vi "DownloadPackageFromNevstopFTP.vi"(8 "error in (no error)":errorcluster, 11 "CommandLine":string[](array[string])) -> (0 "error out":errorcluster, 2 "test details":string, 3 "output to action":string)   [LabVIEW 2014]
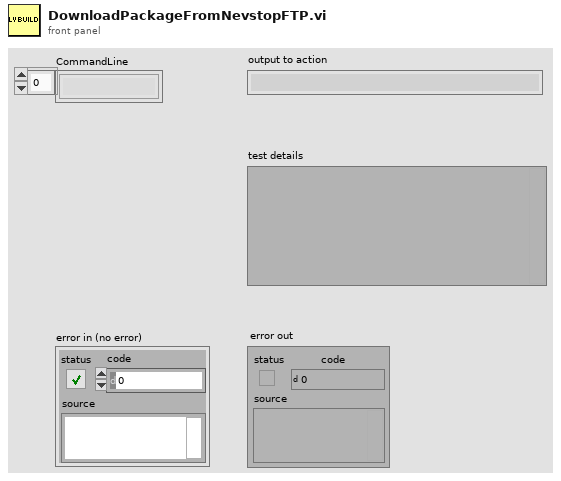
[diagram p1: front panel]
types:
  T1 = cluster{"address":string, "remote port (21)":u16, "userName":string, "passWord":string}
  T2 = typedef "FTP.lvlib/FTP.lvclass/Dir-File Info.ctl" = cluster{"Name":string, "Modify Timestamp":timestamp, "Dir-File Type":T3, "Unique Id":string, "Permissions":string, "Unix Mode":u16, "Owner":string, "Group":string, "FileSize":i64}
  T3 = typedef "FTP.lvlib/FTP.lvclass/Dir-File Type.ctl" = enum16{"File", "Listed Directory", "Parent Directory", "Directory", "Unknown"}
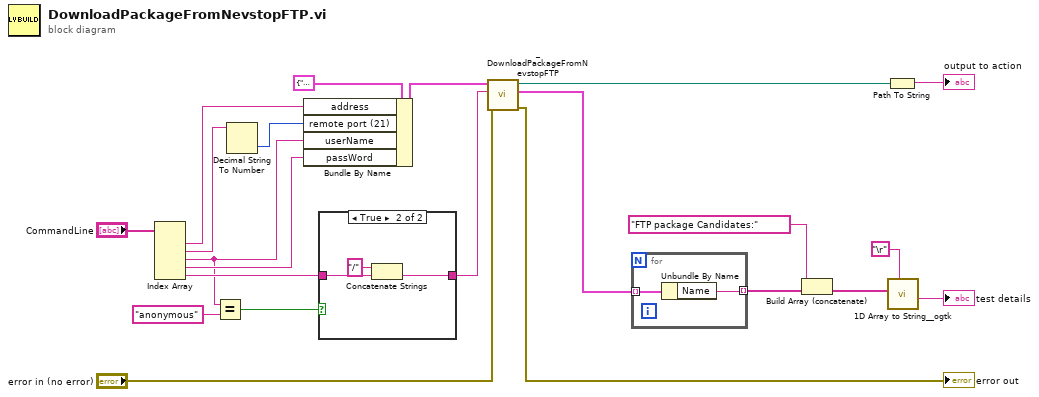
[diagram p0: block diagram]
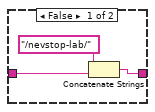
[diagram p2: hidden frame]
diagram:
  n1 = Index Array(array="CommandLine") -> (element #1=w16:string, element #2=w15:string, element #3=w3:string, element #4=w13:string, element #5=w12:string)  [unwired: 5 in]
  n2 = Equal?(x=w3, y="anonymous") -> (x = y?=w1:bool)
  n3 = Decimal String To Number(string=w15) -> (number=w14:i32)  [unwired: 2 in, 1 out]
  n4 = Bundle By Name(cluster=T1 {"address"="vipm.nevstop.top", "remote port (21)"=1986, "userName"="", "passWord"=""} ("ftp"), "address"=w16, "remote port (21)"=w14, "userName"=w3, "passWord"=w13) -> (w17:T1)
  n5 = case shown="True" w1 {
    tunnel: w12 -> [w25 w28]
    tunnel: [w23 w27] -> w11
    frame False {
      n6 = Concatenate Strings("/nevstop-lab/" ("RemoteDirectory"), w25) -> (w23:string)
    }
    frame True {
      n7 = Concatenate Strings("/" ("string"), w28) -> (w27:string)
    }
  }
  n8 = call "_DownloadPackageFromNevstopFTP.vi"("error in (no error)"="error in (no error)", "RemoteDirectory"=w11, "ftp"=w17) -> ("error out"=→"error out":errorcluster, "candidates"=w6:T2[], "localdir"=w8:path)  [unwired: 5 in, 1 out]
  n9 = for {
    tunnel: [w29] -> w21 mode=indexing
    tunnel: w6 -> [w30] mode=indexing
    n10 = Unbundle By Name(w30) -> ("Name"=w29:string)
  }
  n11 = Build Array (concatenate)("FTP package Candidates:" ("Name"), w21) -> (w5:string[])
  n12 = Path To String(path=w8) -> (string=→"output to action":string)
  n13 = call <userlib>:"1D Array to String__ogtk.vi"("delimiter (Tab)"="\r", "Array of Strings"=w5) -> ("delimited string"=→"test details":string)  [unwired: 9 in]
